vi "group channels.vi"(10 "Channels":T4[](array[typedef]) {"Mapping"."VS Reference" format="%.0x"}, 11 "Item Ref in":T1 format="%.0x") -> (2 "Groups":T2[](array[typedef]) {"Channel Data"."Mapping"."VS Reference" format="%.0x"}, 3 "Item Ref out":T1 format="%.0x")   [LabVIEW 2021, in "Modbus Master System Explorer.lvlib"]
uses:
  Modbus Master System Explorer.lvlib
  Shared/Controls/Data Model/Channel.ctl
  Modbus Type.ctl
  <vilib>/NI VeriStand/Custom Device API/Custom Device Channel Type.ctl
  Shared/Controls/Data Model/Mapping.ctl
  Shared/Controls/Data Model/DataType.ctl
  <vilib>/NI VeriStand/Custom Device API/Custom Device Item Ref.ctl
  Engine/SubVIs/Bulk Data Access.ctl
  <vilib>/NI VeriStand/Custom Device API/Custom Device API.lvlib
  Shared/Modbus Master Shared.lvlib
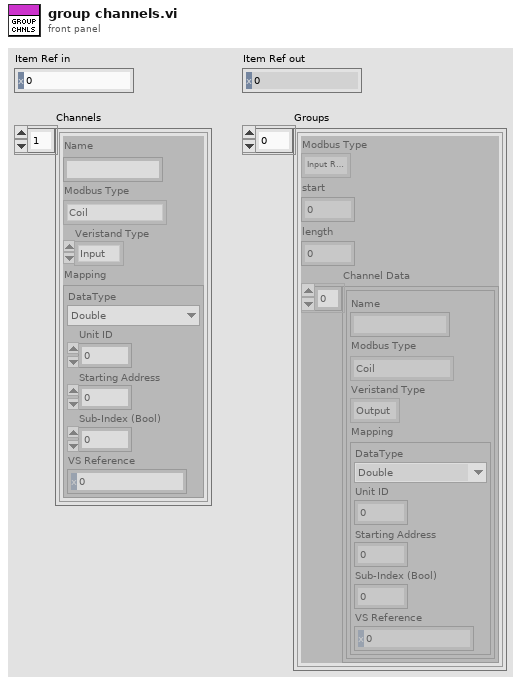
[diagram p1: front panel]
types:
  T1 = typedef "Custom Device API.lvlib/Custom Device Item Ref.ctl" = u64
  T2 = typedef "Modbus Master Shared.lvlib/Bulk Data Access.ctl" = cluster{"Modbus Type":T3, "start":u16, "length":u16, "Channel Data":T4[]}
  T3 = typedef "Modbus Master Shared.lvlib/Modbus Type.ctl" = enum16{"Coil", "Discrete Input", "Holding Register", "Input Register"}
  T4 = typedef "Modbus Master Shared.lvlib/Channel.ctl" = cluster{"Name":string, "Modbus Type":T3, "Veristand Type":T5, "Mapping":T6}
  T5 = typedef "Custom Device API.lvlib/Custom Device Channel Type.ctl" = enum16{"Input", "Output"}
  T6 = typedef "Modbus Master Shared.lvlib/Mapping.ctl" = cluster{"DataType":T7, "Unit ID":u8, "Starting Address":u16, "Sub-Index (Bool)":u16, "VS Reference":T1}
  T7 = typedef "Modbus Master Shared.lvlib/DataType.ctl" = enum16{"Double", "Single", "I64", "I32", "I16", "I8", "U64", "U32", "U16", "U8", "Boolean"}
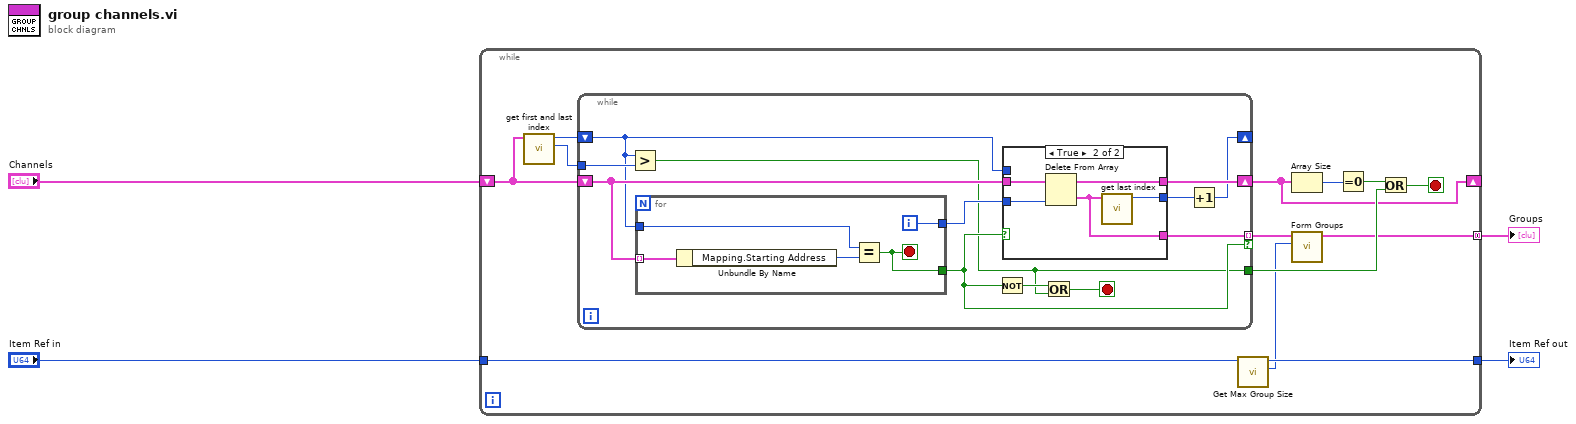
[diagram p0: block diagram]
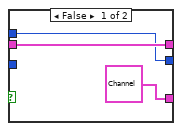
[diagram p2: hidden frame]
diagram:
  n1 = while {
    tunnel: [w8] -> w4 mode=concatenating
    shift-right: [w10] -> _
    shift-left: "Channels" -> [w16]
    tunnel: "Item Ref in" -> [w7]
    tunnel: [w6] -> w2
    stop <- w11 stop-if-true
    n2 = call "get first and last index.vi"("Channels In"=w16) -> ("Last Register"=w15:i32, "Starting Register"=w17:u16)  [unwired: 8 in, 1 out]
    n3 = while {
      tunnel: w15 -> [w29]
      shift-right: [w23] -> _
      shift-left: w17 -> [w25]
      shift-right: [w26] -> w10
      shift-left: w16 -> [w28]
      tunnel: [w22] -> w9 mode=indexing if=w21
      tunnel: [w18] -> w12
      stop <- w19 stop-if-true
      n4 = Greater?(x=w25, y=w29) -> (0:w18:bool)
      n5 = for {
        tunnel: w28 -> [w40] mode=indexing
        tunnel: [w39] -> w27
        tunnel: [w38] -> w21
        tunnel: w25 -> [w42]
        i -> [w39]
        stop <- w38 stop-if-true
        n6 = Unbundle By Name(w40) -> ("Mapping.Starting Address"=w41:u16)
        n7 = Equal?(x=w42, y=w41) -> (x = y?=w38:bool)
      }
      n8 = Not(x=w21) -> (.not. x?=w20:bool)
      n9 = case shown="True" w21 {
        tunnel: w28 -> [w32 w37]
        tunnel: w27 -> [_ w36]
        tunnel: [w32 w35] -> w26
        tunnel: w25 -> [w31 _]
        tunnel: [w31 w33] -> w24
        tunnel: [T4 {"Name"="", "Modbus Type"=enum."Input Register", "Veristand Type"=enum."Output", "Mapping"={"DataType"=enum."Double", "Unit ID"=0, "Starting Address"=0, "Sub-Index (Bool)"=0, "VS Reference"=0}} ("Channel") w34] -> w22
        frame False {
        }
        frame True {
          n10 = Delete From Array(array=w37, index=w36) -> (deleted portion=w34:T4, array with subset deleted=w35:T4[])  [unwired: 1 in]
          n11 = call "get last index.vi"("Channel"=w34) -> ("Last Index"=w33:u16)  [unwired: 10 in]
        }
      }
      n12 = Or(x=w20, y=w18) -> (x .or. y?=w19:bool)
      n13 = Increment(x=w24) -> (x+1=w23:u16)
    }
    n14 = call "Get Max Group Size.vi"("Item Ref in"=w7) -> ("Value"=w5:i32, "Item Ref out"=w6:T1)  [unwired: 8 in, 1 out]
    n15 = Array Size(array=w10) -> (size(s)=w14:i32)
    n16 = call "Form Groups.vi"("Max Size in"=w5, "Array in"=w9) -> ("Array out"=w8:T2[])  [unwired: 9 in]
    n17 = Equal To 0?(x=w14) -> (x = 0?=w13:bool)
    n18 = Or(x=w13, y=w12) -> (x .or. y?=w11:bool)
  }
  "Groups" <- w4
  "Item Ref out" <- w2
